vi "setUp.vi"(8 "error in (no error)":errorcluster, 11 "FrameworkSubTestSuite in":refnum<class "FrameworkSubTestSuite.lvclass">) -> (0 "error out":errorcluster, 3 "FrameworkSubTestSuite out":refnum<class "FrameworkSubTestSuite.lvclass">)   [LabVIEW 2013, in "FrameworkSubTestSuite.lvclass"]
uses:
  FrameworkSubTestSuite.lvclass
  Classes/TestSuite/TestSuite.lvclass
panel:
  out "created new?":bool
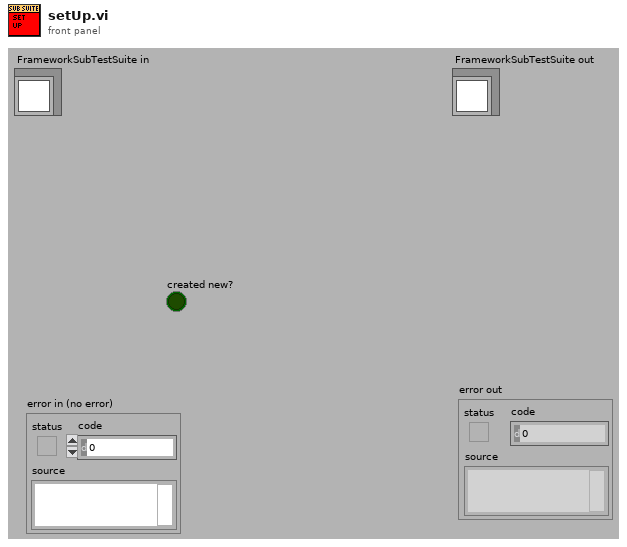
[diagram p1: front panel]
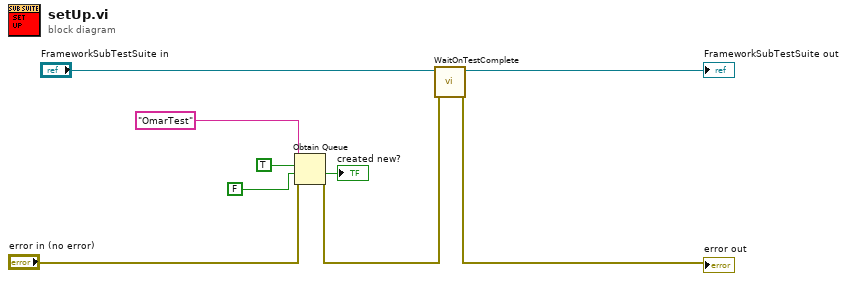
[diagram p0: block diagram]
diagram:
  n1 = Obtain Queue(name (unnamed)="OmarTest", element data type=TRUE, create if not found? (T)=FALSE, error in (no error)="error in (no error)") -> (created new?=→"created new?":bool, error out=w4:errorcluster)  [unwired: 1 in, 1 out]
  n2 = call "WaitOnTestComplete.vi"("error in (no error)"=w4, "TestSuite in"="FrameworkSubTestSuite in") -> ("error out"=→"error out":errorcluster, "TestSuite out"=→"FrameworkSubTestSuite out":refnum<class "FrameworkSubTestSuite.lvclass">)  [unwired: 8 in]
